vi "custom scale test - init.vi"() -> ()   [LabVIEW 2013]
uses:
  <vilib>/DAQmx/read.llb/DAQmx Read.vi
  <vilib>/DAQmx/read.llb/DAQmx Read (Analog 1D Wfm NChan NSamp).vi
  <vilib>/DAQmx/create/channels.llb/DAQmx Create Channel (AI-Current-Basic).vi
  <vilib>/DAQmx/configure/timing.llb/DAQmx Timing (Sample Clock).vi
  <vilib>/DAQmx/create/scale.llb/DAQmx Create Scale (Linear).vi
  <vilib>/DAQmx/miscellaneous.llb/DAQmx Fill In Error Info.vi
  <resource>/objmgr/daqmx.rc
panel:
  out "data":waveform(dbl)[](graph)
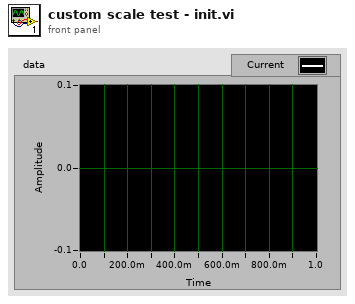
[diagram p1: front panel]
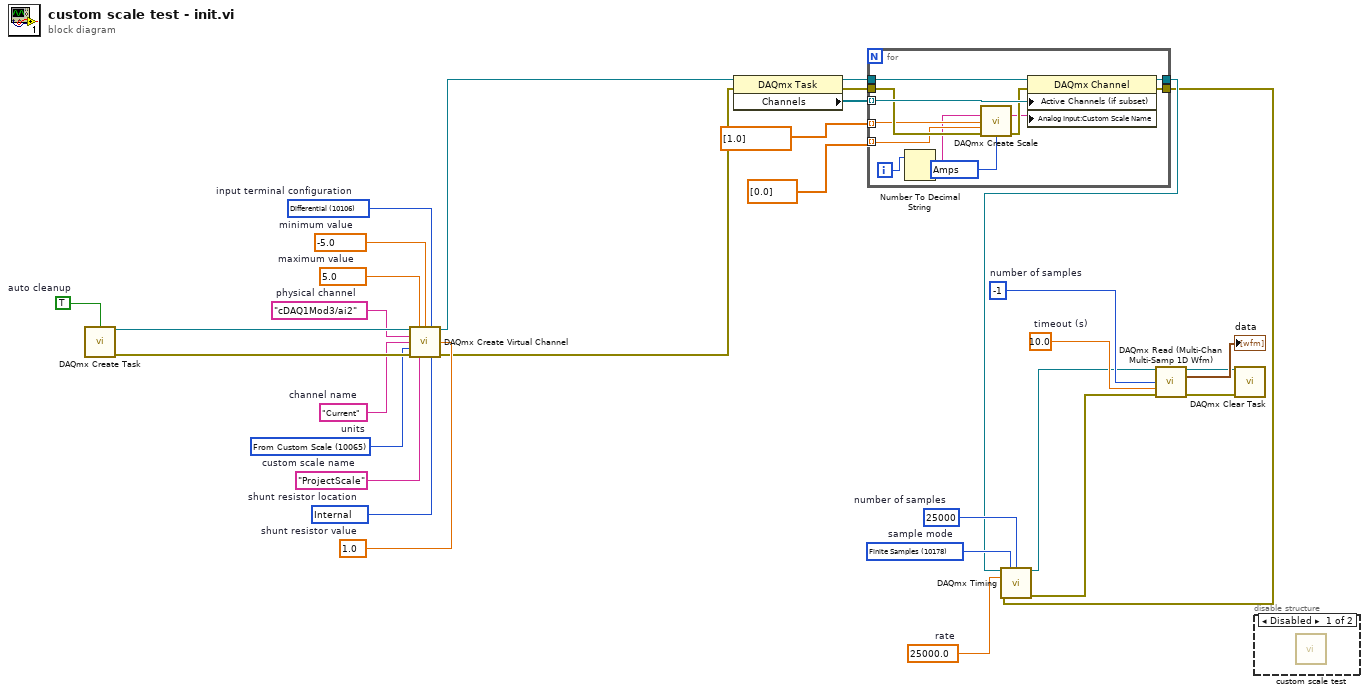
[diagram p0: block diagram]
diagram:
  w12 = 10178 items=["Finite Samples"=10178, "Continuous Samples"=10123, "Hardware Timed Single Point"=12522]  # sample mode
  w13 = 25000  # number of samples
  w14 = 25000.0  # rate
  w15 = 10106 items=["default"=-1, "RSE"=10083, "NRSE"=10078, "Differential"=10106, "Pseudodifferential"=12529]  # input terminal configuration
  w16 = 10065 items=["Amps"=10342, "From Custom Scale"=10065]  # units
  w17 = 1.0  # shunt resistor value
  w18 = 10200 items=["Internal"=10200, "External"=10167]  # shunt resistor location
  w19 = "Current"  # channel name
  w20 = "ProjectScale"  # custom scale name
  w21 = -5.0  # minimum value
  w22 = 5.0  # maximum value
  w23 = "cDAQ1Mod3/ai2"  # physical channel
  w25 = TRUE  # auto cleanup
  w29 = 10.0  # timeout (s)
  w30 = -1  # number of samples
  n1 = call <vilib>:"DAQmx Create Task.vi"("auto cleanup"=w25) -> ("task out"=w24:refnum<k21>, "error out"=w26:errorcluster)  [unwired: 13 in]
  n2 = call-poly <vilib>:"DAQmx Create Virtual Channel.vi"("task in"=w24, "maximum value"=w22, "minimum value"=w21, "input terminal configuration"=w15, "physical channels"=w23, "name to assign"=w19, "external shunt resistor value"=w17, "units"=w16, "error in"=w26, "custom scale name"=w20, "shunt resistor location"=w18) -> ("task out"=w6:refnum<k21>, "error out"=w5:errorcluster)  [unwired: 3 in]
  n3 = property class="DAQmx Task"(reference=w6, error in=w5) -> (reference out=w9:refnum<k21>, error out=w7:errorcluster, "Channels"=w8:refnum<k21>[])
  n4 = for {
    tunnel: w9 -> [w43]
    tunnel: w8 -> [w40] mode=indexing
    tunnel: w7 -> [w39]
    tunnel: [w42] -> w4
    tunnel: [w41] -> w3
    tunnel: dbl[] [0.0] ("Y-Intercept") -> [w36] mode=indexing
    tunnel: dbl[] [1.0] ("Slope") -> [w37] mode=indexing
    i -> [w34]
    w32 = 10342 items=["Volts"=10348, "Amps"=10342, "Deg F"=10144, "Deg C"=10143, "Deg R"=10145, "Kelvins"=10325, "Strain"=10299, "Ohms"=10384, "Hz"=10373, "Seconds"=10364, "Meters"=10219, "Inches"=10379, "Degrees"=10146, "Radians"=10273, "Ticks"=10304, "g"=10186, "m/s^2"=12470, "m/s"=15959, "in/s"=15960, "Pascals"=10081, "Newtons"=15875, "Pounds"=15876, "kgf"=15877, "psi"=15879, "bar"=15880, "Nm"=15881, "oz-in"=15882, "lb-in"=15883, "lb-ft"=15884, "Volts/Volt"=15896, "mVolts/Volt"=15897, "From TEDS"=12516] ("pre-scaled units")
    n5 = Number To Decimal String(number=w34) -> (decimal integer string=w33:string)  [unwired: 1 in]
    n6 = call-poly <vilib>:"DAQmx Create Scale.vi"("name"=w33, "slope"=w37, "y-intercept"=w36, "error in"=w39, "pre-scaled units"=w32) -> ("scale out"=w35:tag, "error out"=w38:errorcluster)  [unwired: 9 in]
    n7 = property class="DAQmx Channel"(reference=w43, error in=w38, "Active Channels (if subset)"=w40, "Analog Input:Custom Scale Name"=w35) -> (reference out=w42:refnum<k21>, error out=w41:errorcluster)
  }
  n8 = call-poly <vilib>:"DAQmx Timing.vi"("task/channels in"=w4, "sample mode"=w12, "samples per channel"=w13, "rate"=w14, "error in"=w3) -> ("task out"=w11:refnum<k21>, "error out"=w10:errorcluster)  [unwired: 9 in]
  n9 = call-poly "DAQmx Read (Multi-Chan Multi-Samp 1D Wfm).vi"("task/channels in"=w11, "number of samples per channel"=w30, "timeout"=w29, "error in"=w10) -> ("task out"=w27:refnum<k21>, "data"=→"data":waveform(dbl)[], "error out"=w28:errorcluster)  [unwired: 9 in]
  n10 = call <vilib>:"DAQmx Clear Task.vi"("task in"=w27, "error in"=w28) -> ()  [unwired: 13 in, 1 out]
  n11 = disable-structure shown="Disabled" {
    frame Disabled {
      n12 = call "custom scale test.vi"() -> ()  [unwired: 10 in, 2 out]
    }
    frame Enabled {
    }
  }
